vi "Init UIMsg Callbacks.vi"(8 "error in (no error)":errorcluster, 11 "SequenceViewPanel in":refnum<class "SequenceViewPanel.lvclass">) -> (0 "error out":errorcluster, 3 "SequenceViewPanel out":refnum<class "SequenceViewPanel.lvclass">)   [LabVIEW 2020, in "TSnax UI.lvlib" / "SequenceViewPanel.lvclass"]
uses:
  SequenceViewPanel.lvclass
  SequenceViewPanel.lvclass/SequenceViewPanel.ctl
  UIMsg Callback.vi
  TSnax/Engine/Engine.lvclass
  TSnax/UIMessage/UIMessage.lvclass
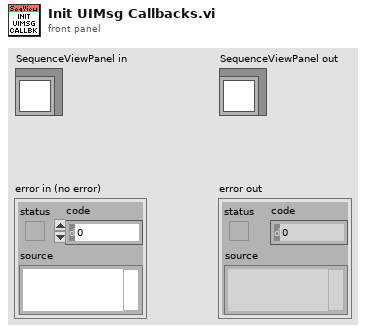
[diagram p1: front panel]
types:
  T1 = typedef "TSnax.lvlib/UIMsg.ctl" = enum16{"Unknown", "BreakOnUserRequest", "BreakOnBreakpoint", "BreakOnRunTimeError", "Trace", "TerminatingExecution", "AbortingExecution", "KillingExecutionThreads", "EndExecution", "ShutDownComplete", "StartExecution", "ProgressPercent", "ProgressText", "StartInteractiveExecution", "EndInteractiveExecution", "TerminatingInteractiveExecution", "TerminationCancelled", "ResumeFromBreak", "StartFileExecution", "EndFileExecution", "ShutDownCancelled", "LocalizationSettingChanged", "OpenWindows", "TileWindows", "CascadeWindows", "ReportChanged", "CloseWindows", "RefreshWindows", "ClientFileChanged", "DisplayReport", "ModelState_Initializing", "ModelState_Waiting", "ModelState_Identified", "ModelState_BeginTesting", "ModelState_TestingComplete", "ModelState_PostProcessingComplete", "ModelState_EnabledStateSet", "ReportLocationChanged", "GotoLocation", "PushUndoItem", "OutputMessages", "TypePaletteFileListChanged", "NonTerminatingThreadsArePreventingTermination", "ModelState_PostProcessing", "ReportCollectionChanged", "RuntimeError"}
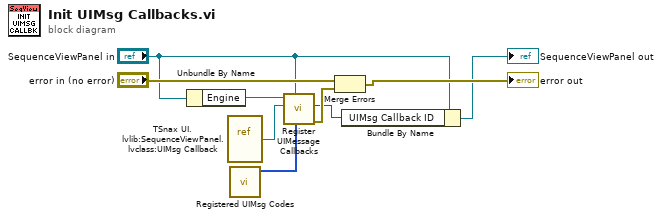
[diagram p0: block diagram]
diagram:
  n1 = Unbundle By Name("SequenceViewPanel in") -> ("Engine"=w1:refnum<class "Engine.lvclass">)
  n2 = vi-ref "TSnax UI.lvlib:SequenceViewPanel.lvclass:UIMsg Callback.vi"() -> (w6:refnum<vi>)
  n3 = call "Registered UIMsg Codes.vi"() -> ("UIMessage IDs"=w5:T1[])  [unwired: 11 in]
  n4 = call "Register UIMessage Callbacks.vi"("UIMessage IDs"=w5, "Owner"="SequenceViewPanel in", "Callback"=w6, "Engine in"=w1) -> ("error out"=w4:errorcluster, "Callback ID"=w3:i32)  [unwired: 5 in, 1 out]
  n5 = Merge Errors("error in (no error)", w4) -> (→"error out":errorcluster)
  n6 = Bundle By Name(cluster="SequenceViewPanel in", "UIMsg Callback ID"=w3) -> (→"SequenceViewPanel out":refnum<class "SequenceViewPanel.lvclass">)
